vi "pulse input 1.vi"() -> ()   [LabVIEW 2023]
uses:
  <vilib>/DAQmx/read.llb/DAQmx Read (Analog Wfm 1Chan NSamp).vi
  <vilib>/DAQmx/write.llb/DAQmx Write (Analog Wfm 1Chan NSamp).vi
  <vilib>/DAQmx/create/channels.llb/DAQmx Create Channel (AI-Voltage-Basic).vi
  <vilib>/DAQmx/configure/timing.llb/DAQmx Timing (Sample Clock).vi
  <vilib>/DAQmx/create/channels.llb/DAQmx Create Channel (AO-Voltage-Basic).vi
  <vilib>/DAQmx/miscellaneous.llb/DAQmx Fill In Error Info.vi
panel:
  out "Duty Cycle 2":dbl
  out "Period 2":dbl
  out "Frequency 2":dbl
  out "Duty Cycle":dbl
  out "Period":dbl
  out "Frequency":dbl
  out "Waveform Graph":waveform(dbl)(graph)
  in  "stop":bool
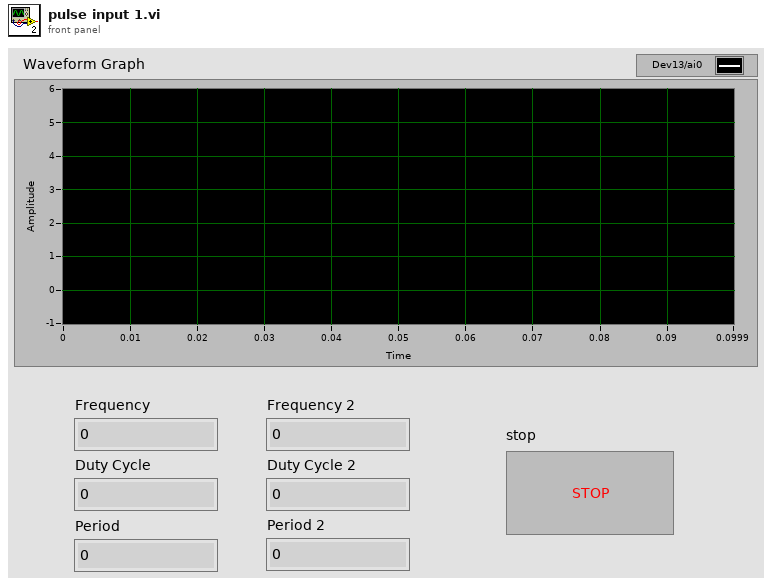
[diagram p1: front panel]
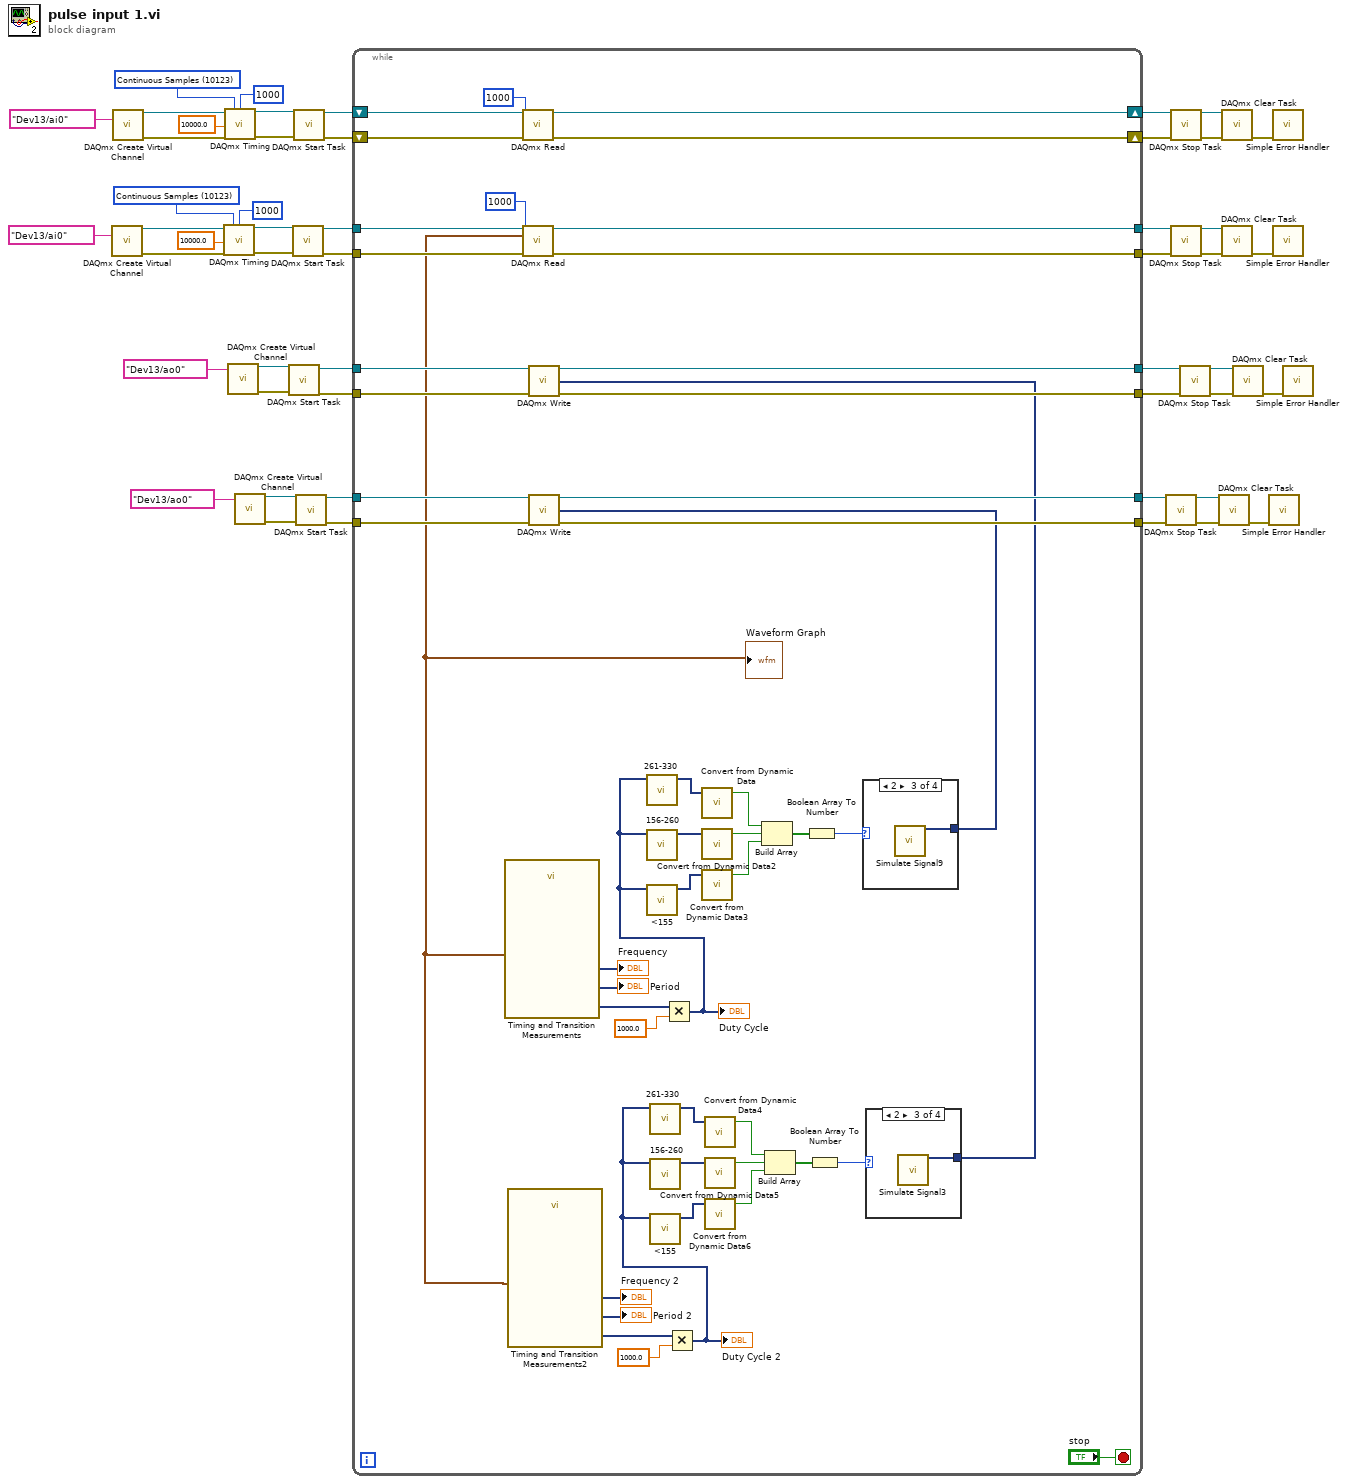
[diagram p0: block diagram]
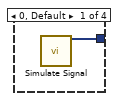
[diagram p2: hidden frame]
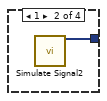
[diagram p3: hidden frame]
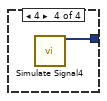
[diagram p4: hidden frame]
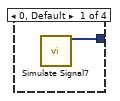
[diagram p5: hidden frame]
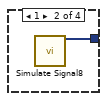
[diagram p6: hidden frame]
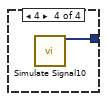
[diagram p7: hidden frame]
diagram:
  w20 = 10123 items=["Finite Samples"=10178, "Continuous Samples"=10123, "Hardware Timed Single Point"=12522] ("sample mode")
  w38 = 10123 items=["Finite Samples"=10178, "Continuous Samples"=10123, "Hardware Timed Single Point"=12522] ("sample mode")
  n1 = call-poly <vilib>:"DAQmx Create Virtual Channel.vi"("physical channels"=tag "Dev13/ai0") -> ("task out"=w25:refnum<k21>, "error out"=w24:errorcluster)  [unwired: 13 in]
  n2 = call-poly <vilib>:"DAQmx Create Virtual Channel.vi"("physical channels"=tag "Dev13/ai0") -> ("task out"=w43:refnum<k21>, "error out"=w42:errorcluster)  [unwired: 13 in]
  n3 = call-poly <vilib>:"DAQmx Timing.vi"("task/channels in"=w25, "sample mode"=w20, "samples per channel"=1000, "rate"=10000.0, "error in"=w24) -> ("task out"=w22:refnum<k21>, "error out"=w23:errorcluster)  [unwired: 9 in]
  n4 = call-poly <vilib>:"DAQmx Timing.vi"("task/channels in"=w43, "sample mode"=w38, "samples per channel"=1000, "rate"=10000.0, "error in"=w42) -> ("task out"=w40:refnum<k21>, "error out"=w41:errorcluster)  [unwired: 9 in]
  n5 = call-poly <vilib>:"DAQmx Create Virtual Channel.vi"("physical channels"=tag "Dev13/ao0") -> ("task out"=w10:refnum<k21>, "error out"=w9:errorcluster)  [unwired: 13 in]
  n6 = call-poly <vilib>:"DAQmx Create Virtual Channel.vi"("physical channels"=tag "Dev13/ao0") -> ("task out"=w35:refnum<k21>, "error out"=w33:errorcluster)  [unwired: 13 in]
  n7 = call <vilib>:"DAQmx Start Task.vi"("task/channels in"=w10, "error in"=w9) -> ("task out"=w4:refnum<k21>, "error out"=w2:errorcluster)  [unwired: 12 in]
  n8 = call <vilib>:"DAQmx Start Task.vi"("task/channels in"=w22, "error in"=w23) -> ("task out"=w17:refnum<k21>, "error out"=w16:errorcluster)  [unwired: 12 in]
  n9 = call <vilib>:"DAQmx Start Task.vi"("task/channels in"=w40, "error in"=w41) -> ("task out"=w50:refnum<k21>, "error out"=w46:errorcluster)  [unwired: 12 in]
  n10 = call <vilib>:"DAQmx Start Task.vi"("task/channels in"=w35, "error in"=w33) -> ("task out"=w34:refnum<k21>, "error out"=w32:errorcluster)  [unwired: 12 in]
  n11 = while {
    shift-right: [w95] -> w49
    shift-left: w50 -> [w98]
    shift-right: [w96] -> w45
    shift-left: w46 -> [w97]
    tunnel: w34 -> [w91]
    tunnel: w32 -> [w90]
    tunnel: [w89] -> w31
    tunnel: [w88] -> w30
    tunnel: w17 -> [w75]
    tunnel: w16 -> [w74]
    tunnel: [w73] -> w12
    tunnel: [w72] -> w11
    tunnel: w4 -> [w58]
    tunnel: [w57] -> w3
    tunnel: w2 -> [w56]
    tunnel: [w55] -> w1
    stop <- "stop" stop-if-true
    n12 = call-poly <vilib>:"DAQmx Read.vi"("task/channels in"=w98, "number of samples per channel"=1000, "error in"=w97) -> ("task out"=w95:refnum<k21>, "error out"=w96:errorcluster)  [unwired: 10 in, 1 out]
    n13 = call-poly <vilib>:"DAQmx Read.vi"("task/channels in"=w75, "number of samples per channel"=1000, "error in"=w74) -> ("task out"=w73:refnum<k21>, "data"=w52:waveform(dbl), "error out"=w72:errorcluster)  [unwired: 10 in]
    "Waveform Graph" <- w52
    n14 = call "Timing and Transition Measurements"("Signals"=w52) -> ("Frequency"=→"Frequency":dynamicdata, "Period"=→"Period":dynamicdata, "Duty Cycle"=w87:dynamicdata)  [unwired: 7 in, 1 out]
    n15 = call "Timing and Transition Measurements2"("Signals"=w52) -> ("Frequency"=→"Frequency 2":dynamicdata, "Period"=→"Period 2":dynamicdata, "Duty Cycle"=w69:dynamicdata)  [unwired: 7 in, 1 out]
    n16 = Multiply(x=w87, y=1000.0) -> (x*y=w85:dynamicdata)
    "Duty Cycle" <- w85
    n17 = call "261-330"("Operand 1"=w85) -> ("Result"=w84:dynamicdata)  [unwired: 9 in, 1 out]
    n18 = call "156-260"("Operand 1"=w85) -> ("Result"=w83:dynamicdata)  [unwired: 9 in, 1 out]
    n19 = call "<155"("Operand 1"=w85) -> ("Result"=w82:dynamicdata)  [unwired: 9 in, 1 out]
    n20 = Multiply(x=w69, y=1000.0) -> (x*y=w67:dynamicdata)
    "Duty Cycle 2" <- w67
    n21 = call "261-330"("Operand 1"=w67) -> ("Result"=w66:dynamicdata)  [unwired: 9 in, 1 out]
    n22 = call "156-260"("Operand 1"=w67) -> ("Result"=w65:dynamicdata)  [unwired: 9 in, 1 out]
    n23 = call "<155"("Operand 1"=w67) -> ("Result"=w64:dynamicdata)  [unwired: 9 in, 1 out]
    n24 = call "Convert from Dynamic Data"("Dynamic Data Type"=w84) -> ("Scalar"=w80:bool)  [unwired: 3 in]
    n25 = call "Convert from Dynamic Data2"("Dynamic Data Type"=w83) -> ("Scalar"=w81:bool)  [unwired: 3 in]
    n26 = call "Convert from Dynamic Data3"("Dynamic Data Type"=w82) -> ("Scalar"=w79:bool)  [unwired: 3 in]
    n27 = call "Convert from Dynamic Data4"("Dynamic Data Type"=w66) -> ("Scalar"=w62:bool)  [unwired: 3 in]
    n28 = call "Convert from Dynamic Data5"("Dynamic Data Type"=w65) -> ("Scalar"=w63:bool)  [unwired: 3 in]
    n29 = call "Convert from Dynamic Data6"("Dynamic Data Type"=w64) -> ("Scalar"=w61:bool)  [unwired: 3 in]
    n30 = Build Array(w80, w81, w79) -> (w78:bool[])
    n31 = Build Array(w62, w63, w61) -> (w60:bool[])
    n32 = Boolean Array To Number(Boolean array=w78) -> (number=w77:u32)
    n33 = Boolean Array To Number(Boolean array=w60) -> (number=w59:u32)
    n34 = case shown="2" w77 {
      tunnel: [w103 w104 w105 w106] -> w53
      frame 0, Default {
        n35 = call "Simulate Signal7"() -> ("DC"=w103:dynamicdata)  [unwired: 14 in, 1 out]
      }
      frame 1 {
        n36 = call "Simulate Signal8"() -> ("Square"=w104:dynamicdata)  [unwired: 14 in, 1 out]
      }
      frame 2 {
        n37 = call "Simulate Signal9"() -> ("Square"=w105:dynamicdata)  [unwired: 14 in, 1 out]
      }
      frame 4 {
        n38 = call "Simulate Signal10"() -> ("DC"=w106:dynamicdata)  [unwired: 14 in, 1 out]
      }
    }
    n39 = call-poly <vilib>:"DAQmx Write.vi"("task/channels in"=w91, "data"=w53, "error in"=w90) -> ("task out"=w89:refnum<k21>, "error out"=w88:errorcluster)  [unwired: 10 in, 1 out]
    n40 = case shown="2" w59 {
      tunnel: [w99 w100 w101 w102] -> w54
      frame 0, Default {
        n41 = call "Simulate Signal"() -> ("DC"=w99:dynamicdata)  [unwired: 14 in, 1 out]
      }
      frame 1 {
        n42 = call "Simulate Signal2"() -> ("Square"=w100:dynamicdata)  [unwired: 14 in, 1 out]
      }
      frame 2 {
        n43 = call "Simulate Signal3"() -> ("Square"=w101:dynamicdata)  [unwired: 14 in, 1 out]
      }
      frame 4 {
        n44 = call "Simulate Signal4"() -> ("DC"=w102:dynamicdata)  [unwired: 14 in, 1 out]
      }
    }
    n45 = call-poly <vilib>:"DAQmx Write.vi"("task/channels in"=w58, "data"=w54, "error in"=w56) -> ("task out"=w57:refnum<k21>, "error out"=w55:errorcluster)  [unwired: 10 in, 1 out]
  }
  n46 = call <vilib>:"DAQmx Stop Task.vi"("task/channels in"=w31, "error in"=w30) -> ("task out"=w29:refnum<k21>, "error out"=w27:errorcluster)  [unwired: 12 in]
  n47 = call <vilib>:"DAQmx Stop Task.vi"("task/channels in"=w49, "error in"=w45) -> ("task out"=w48:refnum<k21>, "error out"=w44:errorcluster)  [unwired: 12 in]
  n48 = call <vilib>:"DAQmx Stop Task.vi"("task/channels in"=w12, "error in"=w11) -> ("task out"=w15:refnum<k21>, "error out"=w13:errorcluster)  [unwired: 12 in]
  n49 = call <vilib>:"DAQmx Stop Task.vi"("task/channels in"=w3, "error in"=w1) -> ("task out"=w7:refnum<k21>, "error out"=w5:errorcluster)  [unwired: 12 in]
  n50 = call <vilib>:"DAQmx Clear Task.vi"("task in"=w29, "error in"=w27) -> ("error out"=w28:errorcluster)  [unwired: 13 in]
  n51 = call <vilib>:"DAQmx Clear Task.vi"("task in"=w48, "error in"=w44) -> ("error out"=w47:errorcluster)  [unwired: 13 in]
  n52 = call <vilib>:"DAQmx Clear Task.vi"("task in"=w15, "error in"=w13) -> ("error out"=w14:errorcluster)  [unwired: 13 in]
  n53 = call <vilib>:"DAQmx Clear Task.vi"("task in"=w7, "error in"=w5) -> ("error out"=w6:errorcluster)  [unwired: 13 in]
  n54 = call <vilib>:"Simple Error Handler.vi"("error in (no error)"=w28) -> ()  [unwired: 4 in, 5 out]
  n55 = call <vilib>:"Simple Error Handler.vi"("error in (no error)"=w47) -> ()  [unwired: 4 in, 5 out]
  n56 = call <vilib>:"Simple Error Handler.vi"("error in (no error)"=w14) -> ()  [unwired: 4 in, 5 out]
  n57 = call <vilib>:"Simple Error Handler.vi"("error in (no error)"=w6) -> ()  [unwired: 4 in, 5 out]
